vi "Dialog with Timeout_stay_silent.vi"   [LabVIEW 2012]
doc: "Displays a standard dialog box that prompts users to enter information, such as a user name and password.\n--------------------\n\nThis Express VI is configured as follows:\n\nMessage to Display to the User:\nThe inputs are:"
uses:
  THD_Mess_Status.vi
panel:
  # "Sound disturbance detected!!\nPlease be Silent !!!\nMeasurement underway!!"
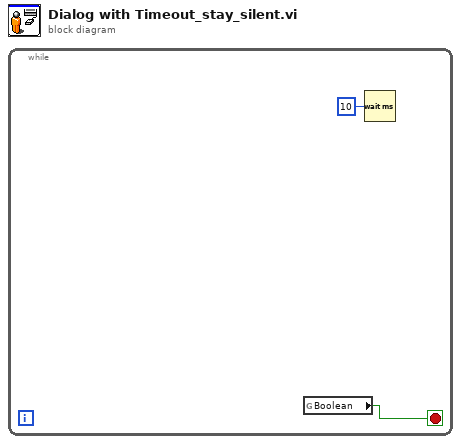
[diagram p0: block diagram]
diagram:
  n1 = while {
    stop <- w1 stop-if-true
    n2 = global read "THD_Mess_Status.vi" "Boolean"() -> (w1:bool)
    n3 = Wait (ms)(milliseconds to wait=u32 10) -> ()  [unwired: 1 out]
  }
